vi "COMPANY -City and State.vi"() -> (1 "Prov|State":string, 3 "City":string)   [LabVIEW 2019]
uses:
  ctlFNCoCustomization.ctl
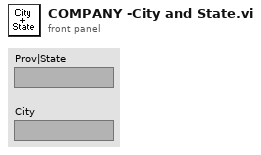
[diagram p1: front panel]
types:
  T1 = typedef "ctlFNCoCustomization.ctl" = enum16{"pre-init", "Init", "Write Co. Info to ini", "GET CFG PARAM", "GET Param Value for Name", "GET ALL"}
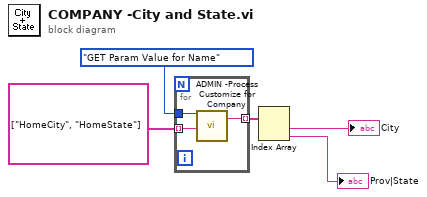
[diagram p0: block diagram]
diagram:
  n1 = for {
    tunnel: ctlFNCoCustomization."GET Param Value for Name" ("SET") -> [w8]
    tunnel: string[] ["HomeCity", "HomeState"] -> [w6] mode=indexing
    tunnel: [w7] -> w3 mode=indexing
    n2 = call "ADMIN -Process Customize for Company.vi"("SET"=w8, "KEY"=w6) -> ("VALUE"=w7:string)  [unwired: 3 in, 14 out]
  }
  n3 = Index Array(array=w3) -> (element #1=→"City":string, element #2=→"Prov|State":string)  [unwired: 2 in]
